vi "capCalc.vi"(5 "capCalcCut":i8, 6 "VolTrig 3":dbl[][](array[numeric]), 7 "capCalc":bool, 8 "Ch4 in":dbl[](array[numeric]), 9 "Ch3 in":dbl[](array[numeric]), 10 "Ch2 in":dbl[](array[numeric]), 11 "Ch1 in":dbl[](array[numeric])) -> (0 "capOut Ch4":dbl format="%0.2f", 1 "capOut Ch3":dbl format="%0.2f", 2 "capOut Ch2":dbl format="%0.2f", 3 "capOut Ch1":dbl format="%0.2f")   [LabVIEW 2021]
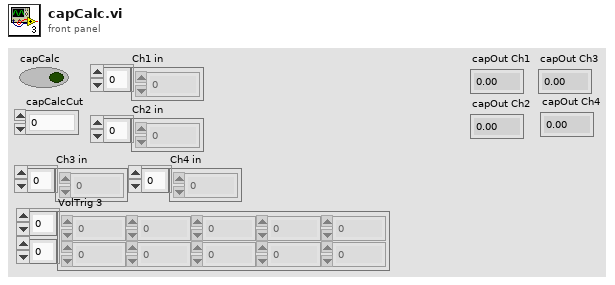
[diagram p1: front panel]
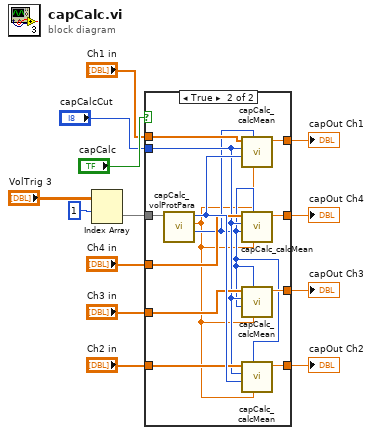
[diagram p0: block diagram]
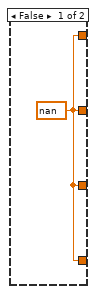
[diagram p2: hidden frame]
diagram:
  n1 = Index Array(array="VolTrig 3", index (row)=1) -> (element=w1:dbl[])  [unwired: 1 in]
  n2 = case shown="True" "capCalc" {
    tunnel: w1 -> [_ w27]
    tunnel: "capCalcCut" -> [_ w17]
    tunnel: [w14 w26] -> w11
    tunnel: "Ch1 in" -> [_ w25]
    tunnel: [w14 w23] -> w10
    tunnel: [w14 w22] -> w9
    tunnel: [w14 w21] -> w8
    tunnel: "Ch3 in" -> [_ w20]
    tunnel: "Ch2 in" -> [_ w19]
    tunnel: "Ch4 in" -> [_ w18]
    frame False {
      w14 = nan
    }
    frame True {
      n3 = call "capCalc_volProtPara.vi"("volProtTri"=w27) -> ("signStart"=w16:i32, "signLength"=w15:dbl, "sigReps"=w24:i32)  [unwired: 8 in]
      n4 = call "capCalc_calcMean.vi"("signLength"=w15, "signStart"=w16, "sigReps"=w24, "capCalcCut"=w17, "Ch in"=w25) -> ("capMeanOut"=w26:dbl)  [unwired: 6 in]
      n5 = call "capCalc_calcMean.vi"("signLength"=w15, "signStart"=w16, "sigReps"=w16, "capCalcCut"=w17, "Ch in"=w18) -> ("capMeanOut"=w21:dbl)  [unwired: 6 in]
      n6 = call "capCalc_calcMean.vi"("signLength"=w15, "signStart"=w16, "sigReps"=w16, "capCalcCut"=w17, "Ch in"=w20) -> ("capMeanOut"=w22:dbl)  [unwired: 6 in]
      n7 = call "capCalc_calcMean.vi"("signLength"=w15, "signStart"=w16, "sigReps"=w24, "capCalcCut"=w17, "Ch in"=w19) -> ("capMeanOut"=w23:dbl)  [unwired: 6 in]
    }
  }
  "capOut Ch1" <- w11
  "capOut Ch2" <- w10
  "capOut Ch3" <- w9
  "capOut Ch4" <- w8
